vi "Recalc Histogram.vi"(11 "Rolling array in":T2) -> (2 "standard deviation":dbl, 3 "Hist and fit":T1(array[cluster]))   [LabVIEW 2016]
uses:
  <vilib>/Analysis/6fits.llb/Curve Fitting Criteria.ctl
  Global Variables/Global Resolution.vi
  <vilib>/Analysis/NI_AALBase.lvlib
  <vilib>/Analysis/NI_AALPro.lvlib
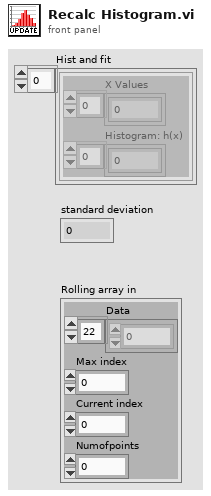
[diagram p1: front panel]
types:
  T1 = cluster{"X Values":dbl[], "Histogram: h(x)":i32[]}[]
  T2 = cluster{"Data":i32[], "Max index":i32, "Current index":i32, "Numofpoints":i32}
  T3 = typedef "NI_AALPro.lvlib/Curve Fitting Criteria.ctl" = u16
  T4 = cluster{"X Values":dbl[], "Histogram: h(x)":i32[]}
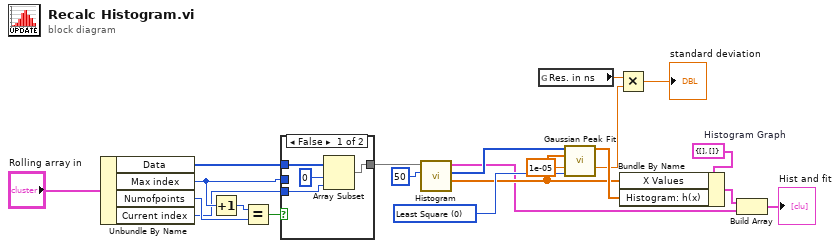
[diagram p0: block diagram]
diagram:
  w9 = T3 0 items=["Least Square", "Least Absolute Residual", "Bisquare"] ("method")
  w12 = T4 {"X Values"=[], "Histogram: h(x)"=[]}  # Histogram Graph
  n1 = Unbundle By Name("Rolling array in") -> ("Data"=w20:i32[], "Max index"=w18:i32, "Numofpoints"=w14:i32, "Current index"=w13:i32)
  n2 = Increment(x=w18) -> (x+1=w17:i32)
  n3 = Equal?(x=w17, y=w14) -> (x = y?=w16:bool)
  n4 = case shown="False" w16 {
    tunnel: w20 -> [w25 w26]
    tunnel: w18 -> [_ _]
    tunnel: [w23 w26] -> w19
    tunnel: w13 -> [w22 _]
    frame False {
      n5 = Array Subset(array=w25, index=0, length=w22) -> (w23:i32[])
    }
    frame True {
    }
  }
  n6 = call <vilib>:"Histogram.vi"("intervals"=50, "X"=w19) -> ("X Values"=w8:dbl[], "Histogram: h(x)"=w7:i32[], "Histogram Graph"=w5:T4)  [unwired: 6 in, 1 out]
  n7 = global read "Global Resolution.vi" "Res. in ns"() -> (w3:ext)
  n8 = call <vilib>:"Gaussian Peak Fit.vi"("Y"=w7, "X"=w8, "tolerance"=1e-05, "method"=w9) -> ("Best Gaussian Fit"=w11:dbl[], "standard deviation"=w2:dbl)  [unwired: 5 in, 5 out]
  n9 = Multiply(x=w3, y=w2) -> (x*y=→"standard deviation":ext)
  n10 = Bundle By Name(cluster=w12, "X Values"=w8, "Histogram: h(x)"=w11) -> (w6:T4)
  n11 = Build Array(w6, w5) -> (→"Hist and fit":T1)
